vi "sub_stream-arr2img.vi"(8 "error in":errorcluster, 11 "imgarr":u8[](array[numeric])) -> (0 "error out":errorcluster, 3 "Image Dst Out":T1)   [LabVIEW 2019]
uses:
  <vilib>/vision/Image Controls.llb/IMAQ Image.ctl
  <vilib>/vision/NI_Vision_Development_Module.lvlib
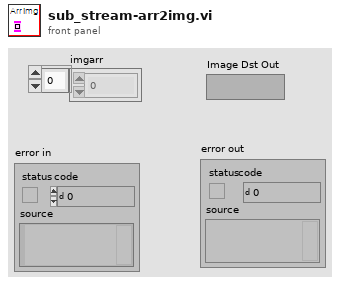
[diagram p1: front panel]
types:
  T1 = typedef "IMAQ Image.ctl" = refnum<image>
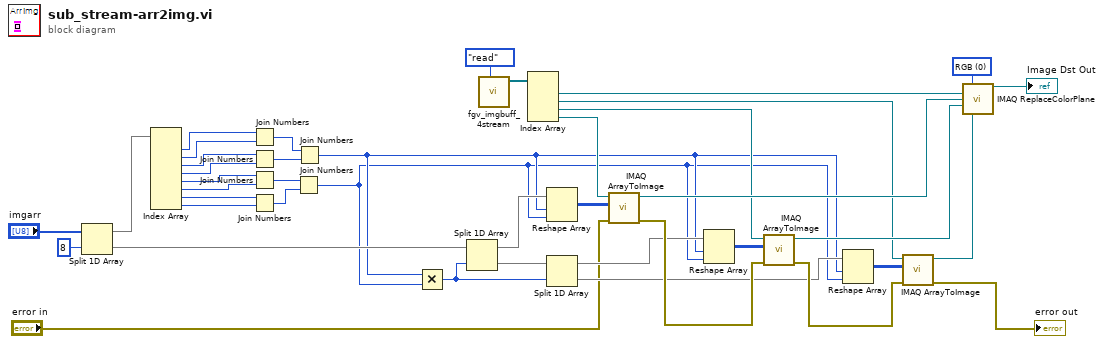
[diagram p0: block diagram]
diagram:
  w40 = u16 0 items=["RGB", "HSL", "HSV", "HSI"] ("Color Mode")
  n1 = Split 1D Array(array="imgarr", index=8 ("인덱스")) -> (first subarray=w3:u8[], second subarray=w35:u8[])
  n2 = Index Array(array=w3) -> (element #1=w13:u8, element #2=w12:u8, element #3=w4:u8, element #4=w5:u8, element #5=w10:u8, element #6=w11:u8, element #7=w15:u8, element #8=w14:u8)  [unwired: 8 in]
  n3 = Join Numbers(hi=w13, lo=w12) -> ((hi.lo)=w7:u16)
  n4 = Join Numbers(hi=w4, lo=w5) -> ((hi.lo)=w6:u16)
  n5 = Join Numbers(hi=w10, lo=w11) -> ((hi.lo)=w9:u16)
  n6 = Join Numbers(hi=w15, lo=w14) -> ((hi.lo)=w8:u16)
  n7 = Join Numbers(hi=w9, lo=w8) -> ((hi.lo)=w1:u32)
  n8 = Join Numbers(hi=w7, lo=w6) -> ((hi.lo)=w2:u32)
  n9 = Multiply(x=w2, y=w1) -> (x*y=w25:u32)
  n10 = Split 1D Array(array=w35, index=w25) -> (first subarray=w28:u8[], second subarray=w41:u8[])
  n11 = call "fgv_imgbuff_4stream.vi"("cmd"=enum16{"cread", "read", "close"}."read") -> ("img out"=w23:T1[])  [unwired: 9 in, 1 out]
  n12 = Index Array(array=w23) -> (element #1=w22:T1, element #2=w21:T1, element #3=w20:T1, element #4=w19:T1)  [unwired: 4 in]
  n13 = Reshape Array(w28, w2, w1) -> (w31:u8[][])
  n14 = Split 1D Array(array=w41, index=w25) -> (first subarray=w27:u8[], second subarray=w26:u8[])
  n15 = call "IMAQ ArrayToImage"("error in (no error)"="error in", "Image Pixels (U8)"=w31, "Image"=w19) -> ("error out"=w34:errorcluster, "Image Out"=w39:T1)  [unwired: 7 in]
  n16 = Reshape Array(w27, w2, w1) -> (w30:u8[][])
  n17 = call "IMAQ ArrayToImage"("error in (no error)"=w34, "Image Pixels (U8)"=w30, "Image"=w20) -> ("error out"=w33:errorcluster, "Image Out"=w38:T1)  [unwired: 7 in]
  n18 = Reshape Array(w26, w2, w1) -> (w29:u8[][])
  n19 = call "IMAQ ArrayToImage"("error in (no error)"=w33, "Image Pixels (U8)"=w29, "Image"=w21) -> ("error out"=→"error out":errorcluster, "Image Out"=w37:T1)  [unwired: 7 in]
  n20 = call "IMAQ ReplaceColorPlane"("Color Mode"=w40, "Image Dst"=w22, "Red or Hue Plane"=w39, "Green or Sat Plane"=w38, "Blue or Luma or Val or Inten Plane"=w37) -> ("Image Dst Out"=→"Image Dst Out":T1)  [unwired: 9 in, 1 out]
